vi "Initialize Hardware.vi"(8 "error in (no error)":errorcluster, 11 "GE Reflective Memory Transceiver in":refnum<class "GE Reflective Memory Transceiver.lvclass">) -> (0 "error out":errorcluster, 3 "GE Reflective Memory Transceiver out":refnum<class "GE Reflective Memory Transceiver.lvclass">)   [LabVIEW 2020, in "GE Reflective Memory.lvlib" / "GE Reflective Memory Transceiver.lvclass"]
uses:
  GE Reflective Memory Transceiver.lvclass
  Driver/Source/Typedefs/GE 5565PIORC.Typedef.DMA Wait Mode.ctl
  GE Reflective Memory Transceiver.lvclass/GE Reflective Memory Transceiver.ctl
  Driver/Source/GE 5565PIORC.lvclass/GE 5565PIORC.ctl
  Driver/Source/Properties/Registers/GE 5565PIORC.Registers.LAS1RR.PCI Address Range.Get.vi
  Driver/Source/Methods/GE 5565PIORC.PXI Interrupts.Enable.vi
  Driver/Source/Properties/Registers/GE 5565PIORC.Registers.DMACSR0.Channel 0 Enable.Set.vi
  Driver/Source/Properties/Registers/GE 5565PIORC.Registers.INTCSR.Local DMA Channel 0 Interrupt Enable.Set.vi
  Driver/Source/Properties/Registers/GE 5565PIORC.Registers.Local Configuration.Read.vi
  Driver/Source/Properties/Registers/GE 5565PIORC.Registers.Local Configuration.Read (U32).vi
  Driver/Source/Properties/Registers/GE 5565PIORC.Registers.Local Configuration.Read (U8).vi
  Driver/Source/Properties/Registers/GE 5565PIORC.Registers.Local Configuration.Write.vi
  Driver/Source/Properties/Registers/GE 5565PIORC.Registers.Local Configuration.Write (U8).vi
  Driver/Source/Methods/GE 5565PIORC.Bit Manipulation.Set Bit.vi
  Driver/Source/Methods/GE 5565PIORC.Bit Manipulation.Set Bit (U8).vi
  Driver/Source/Properties/Registers/GE 5565PIORC.Registers.Local Configuration.Write (U32).vi
  Driver/Source/Methods/GE 5565PIORC.Bit Manipulation.Set Bit (U32).vi
  Driver/Source/Methods/GE 5565PIORC.Registers.Read.vi
  Driver/Source/Methods/GE 5565PIORC.Registers.Read (U32).vi
  Driver/Source/Methods/GE 5565PIORC.Registers.Read (U8).vi
  Driver/Source/Methods/GE 5565PIORC.Registers.Write.vi
  Driver/Source/Methods/GE 5565PIORC.Registers.Write (U8).vi
  Driver/Source/Methods/GE 5565PIORC.Registers.Write (U32).vi
  Driver/Source/GE 5565PIORC.lvclass
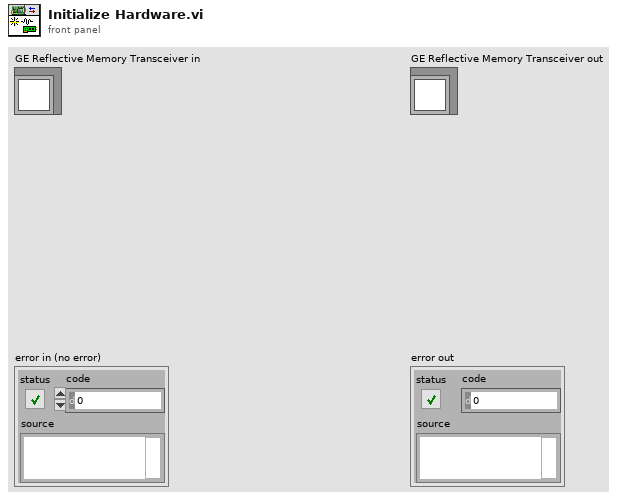
[diagram p1: front panel]
types:
  T1 = typedef "GE 5565PIORC.lvclass/GE 5565PIORC.Typedef.DMA Wait Mode.ctl" = enum16{"Polling", "Interrupt"}
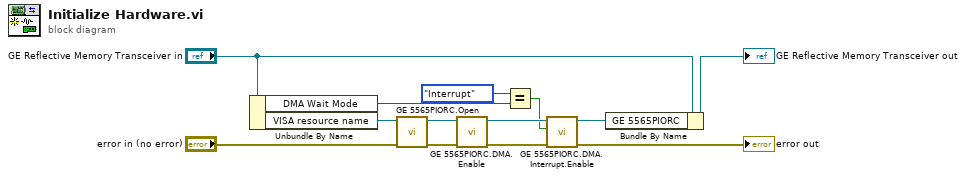
[diagram p0: block diagram]
diagram:
  n1 = Unbundle By Name("GE Reflective Memory Transceiver in") -> ("DMA Wait Mode"=w5:T1, "VISA resource name"=w10:refnum<visa-resource-name>)
  n2 = call "GE 5565PIORC.Open.vi"("error in (no error)"="error in (no error)", "VISA resource name"=w10) -> ("error out"=w9:errorcluster, "GE 5565PIORC"=w8:refnum<class "GE 5565PIORC.lvclass">)  [unwired: 8 in]
  n3 = call "GE 5565PIORC.DMA.Enable.vi"("error in (no error)"=w9, "GE 5565PIORC in"=w8) -> ("error out"=w6:errorcluster, "GE 5565PIORC out"=w7:refnum<class "GE 5565PIORC.lvclass">)  [unwired: 8 in]
  n4 = Equal?(x=GE_5565PIORC.Typedef.DMA_Wait_Mode."Interrupt", y=w5) -> (x = y?=w4:bool)
  n5 = call "GE 5565PIORC.DMA.Interrupt.Enable.vi"("error in (no error)"=w6, "enable (T)"=w4, "GE 5565PIORC in"=w7) -> ("error out"=→"error out":errorcluster, "GE 5565PIORC out"=w1:refnum<class "GE 5565PIORC.lvclass">)  [unwired: 7 in]
  n6 = Bundle By Name(cluster="GE Reflective Memory Transceiver in", "GE 5565PIORC"=w1) -> (→"GE Reflective Memory Transceiver out":refnum<class "GE Reflective Memory Transceiver.lvclass">)
